vi "WaitMsecs - Capture OptoSensor.vi"(8 "error in (no error)":errorcluster, 11 "Wait Msecs":dbl) -> (0 "error out":errorcluster)   [LabVIEW 2013]
uses:
  Test Globals/Global 1.vi
panel:
  out "Intensity Min":i32
  out "Intensity Max":i32
  out "Wavelength Min":i32
  out "Intensity Table":string[](array[string])
  out "Wave Table":string[](array[string])
  out "Wavelength Max":i32=1000
  out "read buffer":string="w=1000 i=4\r\nw=1000 i=4\r\nw=1000 i=4\r\nw=1000 i=4\r\nw=1000 i=4\r\nw=1000 i=4\r\nw=1000 i=4\r\nw=1000 i=4\r\nw=1000 i=4\r\nw=1000 i=4\r\nw=1000 i=4\r\nw=1000 i=4\r\nw=1000 i=4\r\nw=1000 i=4\r\nw=1000 i=4\r\nw=1000 i=4\r\nw=1000 i=4\r\nw=1000 i=4\r\nw=1000 i=4\r\nw=1000 i=4\r\nw=1000 i=4\r\nw=1000 i=4\r\nw=1000 i=4\r\nw=1000 i=4\r\nw=1000 i=4\r\nw=1000 i=4\r\nw=1000 i=4\r\nw=1000 i=4\r\nw=1000 i=4\r\nw=1000 i=4\r\nw=1000 i=4\r\nw=1000 i=4\r\nw=1000 i=4\r\nw=1000 i=4\r\nw=1000 i=4\r\nw=1000 i=4\r\nw=1000 i=4\r\nw=1000 i=4\r\nw=1000 i=4\r\nw=1000 i=4\r\nw=1000 i=4\r\nw=1000 i=4\r\nw=1000 i"
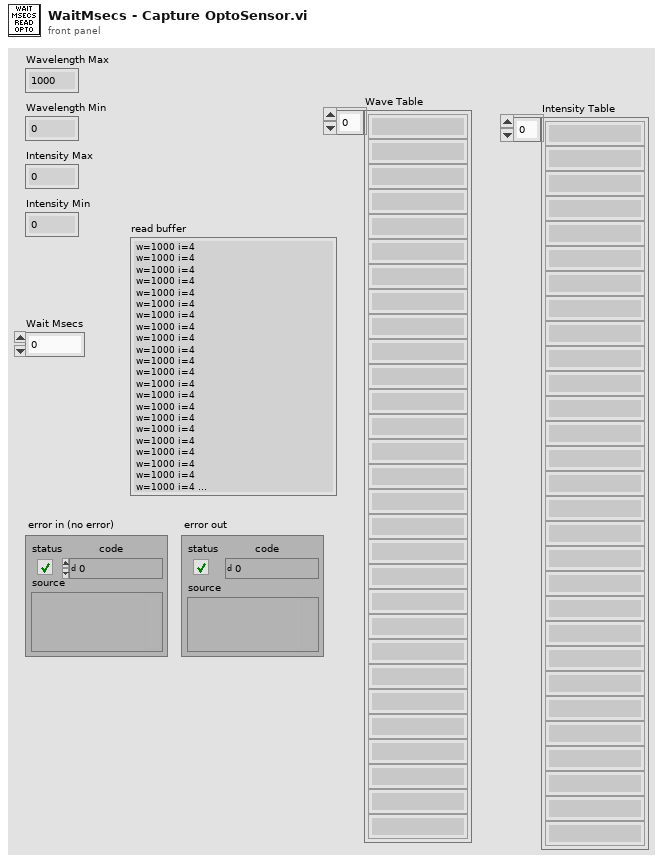
[diagram p1: front panel]
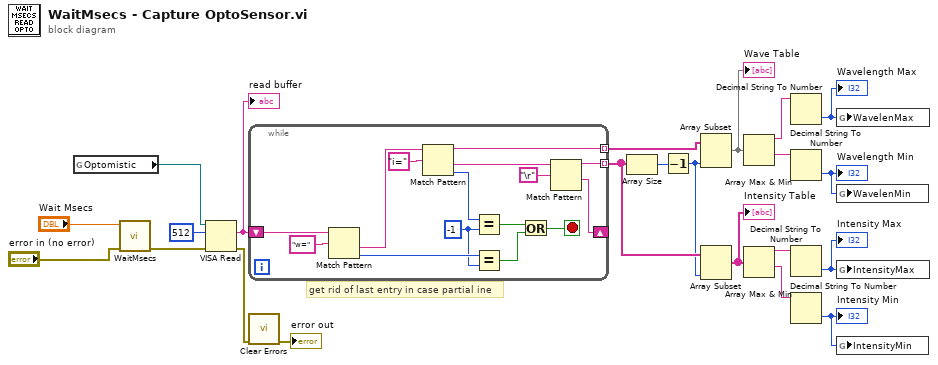
[diagram p0: block diagram]
diagram:
  # "get rid of last entry in case partial ine"
  n1 = global read "Global 1.vi" "Optomistic"() -> (w3:refnum<visa-resource-name>)
  n2 = call "WaitMsecs.vi"("error in (no error)"="error in (no error)", "Wait Msecs"="Wait Msecs") -> ("error out"=w19:errorcluster)  [unwired: 9 in]
  n3 = VISA Read(VISA resource name=w3, byte count=u32 512, error in (no error)=w19) -> (read buffer=w20:string, error out=w2:errorcluster)  [unwired: 2 out]
  "read buffer" <- w20
  n4 = while {
    shift-right: [w23] -> _
    shift-left: w20 -> [w37]
    tunnel: [w27] -> w14 mode=indexing
    tunnel: [w24] -> w11 mode=indexing
    stop <- w28 stop-if-true
    w31 = -1 ("y")
    n5 = Match Pattern(string=w37, regular expression="w=") -> (after substring=w34:string, offset past match=w36:i32)  [unwired: 1 in, 2 out]
    n6 = Match Pattern(string=w34, regular expression="i=") -> (before substring=w27:string, after substring=w26:string, offset past match=w32:i32)  [unwired: 1 in, 1 out]
    n7 = Equal?(x=w32, y=w31) -> (x = y?=w30:bool)
    n8 = Equal?(x=w36, y=w31) -> (x = y?=w29:bool)
    n9 = Or(x=w30, y=w29) -> (x .or. y?=w28:bool)
    n10 = Match Pattern(string=w26, regular expression="\r") -> (before substring=w24:string, after substring=w23:string)  [unwired: 1 in, 2 out]
  }
  n11 = call <vilib>:"Clear Errors.vi"("error in (no error)"=w2) -> ("error out"=→"error out":errorcluster)  [unwired: 6 in]
  n12 = Array Size(array=w11) -> (size(s)=w13:i32)
  n13 = Decrement(x=w13) -> (x-1=w10:i32)
  n14 = Array Subset(array=w14, length=w10) -> (w12:string[])  [unwired: 1 in]
  "Wave Table" <- w12
  n15 = Array Subset(array=w11, length=w10) -> (w9:string[])  [unwired: 1 in]
  "Intensity Table" <- w9
  n16 = Array Max & Min(array=w12) -> (max value=w18:string, min value=w17:string)  [unwired: 2 out]
  n17 = Array Max & Min(array=w9) -> (max value=w16:string, min value=w15:string)  [unwired: 2 out]
  n18 = Decimal String To Number(string=w18) -> (number=w6:i32)  [unwired: 2 in, 1 out]
  "Wavelength Max" <- w6
  n19 = Decimal String To Number(string=w17) -> (number=w5:i32)  [unwired: 2 in, 1 out]
  "Wavelength Min" <- w5
  n20 = Decimal String To Number(string=w16) -> (number=w8:i32)  [unwired: 2 in, 1 out]
  "Intensity Max" <- w8
  n21 = Decimal String To Number(string=w15) -> (number=w7:i32)  [unwired: 2 in, 1 out]
  "Intensity Min" <- w7
  n22 = global write "Global 1.vi" "WavelenMax"(w6) -> ()
  n23 = global write "Global 1.vi" "WavelenMin"(w5) -> ()
  n24 = global write "Global 1.vi" "IntensityMax"(w8) -> ()
  n25 = global write "Global 1.vi" "IntensityMin"(w7) -> ()
